vi "诊断标定3.vi"(8 "CAN端口":u16(ring), 9 "设备索引号":u16(ring), 10 "CAN卡类型":u32(ring)=21) -> ()   [LabVIEW 2013] (continued)
            n809 = property class="VI"(reference=w1301, error in=w1300, "Front Panel.Open"=FALSE ("前面板窗口:打开")) -> ()  [unwired: 2 out]
            n810 = call-poly <vilib>:"Write Key.vi"("section"="总信息", "error in (no error)"=w1293, "value"=w1288, "key"="诊断标定读取地址" ("section"), "refnum"=w1295) -> ("error out"=w1292:errorcluster, "refnum out"=w1291:T25)  [unwired: 4 in, 1 out]
            n811 = call <vilib>:"Close Config Data.vi"("error in (no error)"=w1292, "refnum"=w1291) -> ("error out"=w1290:errorcluster)  [unwired: 8 in, 1 out]
            n812 = call <vilib>:"Clear Errors.vi"("error in (no error)"=w1290) -> ()  [unwired: 6 in, 1 out]
            n813 = local write "强制终止读写标记"(TRUE ("强制终止读写标记")) -> ()
            n814 = local write "停止"(w1299) -> ()
          }
          frame #1 {
            w1307 = u8 0 items=["Normal", "Listen Only"] ("工作方式")
            w1308 = u8 1 items=["Dual Filter", "Single Filter"] ("滤波方式")
            n815 = local read "设备索引号"() -> (w1312:u16)
            n816 = local read "CAN卡类型"() -> (w1313:u32)
            n817 = local read "CAN端口"() -> (w1311:u16)
            n818 = call "CAN_Init-8.6.vi"("CAN卡类型"=w1313, "设备索引号"=w1312, "CAN端口"=w1311, "操作类型"=enum16{"初始化CAN", "关闭CAN"}."初始化CAN", "滤波方式"=w1308, "Accept Code"=u32 0, "簇"=T21 {"打开CAN"=FALSE, "初始化CAN"=TRUE, "开始CAN"=TRUE, "重启"=FALSE, "关闭CAN"=FALSE}, "Mask Code"=u32 4294967295 ("Accept Code"), "工作方式"=w1307, "是否滤波"=FALSE) -> ()  [unwired: 4 in, 6 out]
          }
        }
        n819 = event-data("Discard?"=w1286) -> ()  [unwired: 1 in, 1 out]
      }
      event "终止读写按钮": Value Change {
        n820 = event-data() -> ("NewVal"=w1314:bool)  [unwired: 6 out]
        n821 = case shown="真" w1314 {
          frame False {
          }
          frame True {
            n822 = local write "强制终止读写标记"(TRUE ("强制终止读写标记")) -> ()
          }
        }
      }
      event "1": Value Change {
        w1323 = FALSE ("1")
        n823 = event-data() -> ()  [unwired: 7 out]
        n824 = local write "主板2"(T8."项目信息" ("主从板")) -> ()
        n825 = Not(x=w1323) -> (.not. x?=w1322:bool)
        n826 = local write "1"(w1322) -> ()
        n827 = local write "1 2"(w1323) -> ()
        n828 = local write "1 3"(w1323) -> ()
        n829 = local write "1 4"(w1323) -> ()
        n830 = local write "1 5"(w1323) -> ()
        n831 = local write "1 11"(w1323) -> ()
        n832 = global read "功能码全局.vi" "主板监控2"() -> (w1321:bool[])
        n833 = Index Array(array=w1321, index=6 ("索引")) -> (element=w1316:bool)
        n834 = Select(t=0, s=w1316, f=1) -> (s? t:f=w1317:i32)
        n835 = property on="项目信息" class="Tbl (严格)"("Disabled"=w1317) -> ()  [unwired: 2 in, 2 out]
        n836 = property on="电池实际容量(A)" class="DigNum (严格)"("Disabled"=w1317) -> ()  [unwired: 2 in, 2 out]
        n837 = property on="使用者" class="DigNum (严格)"("Disabled"=w1317) -> ()  [unwired: 2 in, 2 out]
        n838 = property on="SOH(%)" class="DigNum (严格)"("Disabled"=w1317) -> ()  [unwired: 2 in, 2 out]
        n839 = property on="电池额定容量(A)" class="DigNum (严格)"("Disabled"=w1317) -> ()  [unwired: 2 in, 2 out]
        n840 = property on="SOC(%)" class="DigNum (严格)"("Disabled"=w1317) -> ()  [unwired: 2 in, 2 out]
        n841 = property on="项目信息2" class="Clust (严格)"("DisabledEnum"=w1317) -> ()  [unwired: 2 in, 2 out]
        n842 = property on="系统时钟" class="Str"("Disabled"=w1317) -> ()  [unwired: 2 in, 2 out]
        n843 = property on="配置文件版本" class="Str"("Disabled"=w1317) -> ()  [unwired: 2 in, 2 out]
        n844 = property on="车架(牌)号" class="Str"("Disabled"=w1317) -> ()  [unwired: 2 in, 2 out]
        n845 = property on="产品编号" class="Str"("Disabled"=w1317) -> ()  [unwired: 2 in, 2 out]
      }
      event "1 2": Value Change {
        w1334 = FALSE ("1")
        n846 = event-data() -> ()  [unwired: 7 out]
        n847 = local write "主板2"(T8."一级故障阀值" ("主从板")) -> ()
        n848 = Not(x=w1334) -> (.not. x?=w1333:bool)
        n849 = local write "1"(w1334) -> ()
        n850 = local write "1 2"(w1333) -> ()
        n851 = local write "1 3"(w1334) -> ()
        n852 = local write "1 4"(w1334) -> ()
        n853 = local write "1 5"(w1334) -> ()
        n854 = local write "1 11"(w1334) -> ()
        n855 = global read "功能码全局.vi" "主板监控2"() -> (w1332:bool[])
        n856 = Index Array(array=w1332, index=6 ("索引")) -> (element=w1327:bool)
        n857 = Select(t=0, s=w1327, f=1) -> (s? t:f=w1330:i32)
        n858 = property on="一级故障" class="Clust (严格)"("DisabledEnum"=w1330) -> ()  [unwired: 2 in, 2 out]
      }
      event "1 3": Value Change {
        w1345 = FALSE ("1")
        n859 = event-data() -> ()  [unwired: 7 out]
        n860 = local write "主板2"(T8."二级故障阀值" ("主从板")) -> ()
        n861 = Not(x=w1345) -> (.not. x?=w1344:bool)
        n862 = local write "1"(w1345) -> ()
        n863 = local write "1 2"(w1345) -> ()
        n864 = local write "1 3"(w1344) -> ()
        n865 = local write "1 4"(w1345) -> ()
        n866 = local write "1 5"(w1345) -> ()
        n867 = local write "1 11"(w1345) -> ()
        n868 = global read "功能码全局.vi" "主板监控2"() -> (w1343:bool[])
        n869 = Index Array(array=w1343, index=6 ("索引")) -> (element=w1339:bool)
        n870 = Select(t=0, s=w1339, f=1) -> (s? t:f=w1338:i32)
        n871 = property on="一级故障 2" class="Clust (严格)"("DisabledEnum"=w1338) -> ()  [unwired: 2 in, 2 out]
      }
      event "1 4": Value Change {
        w1356 = FALSE ("1")
        n872 = event-data() -> ()  [unwired: 7 out]
        n873 = local write "主板2"(T8."三级故障阀值" ("主从板")) -> ()
        n874 = Not(x=w1356) -> (.not. x?=w1355:bool)
        n875 = local write "1"(w1356) -> ()
        n876 = local write "1 2"(w1356) -> ()
        n877 = local write "1 3"(w1356) -> ()
        n878 = local write "1 4"(w1355) -> ()
        n879 = local write "1 5"(w1356) -> ()
        n880 = local write "1 11"(w1356) -> ()
        n881 = global read "功能码全局.vi" "主板监控2"() -> (w1354:bool[])
        n882 = Index Array(array=w1354, index=6 ("索引")) -> (element=w1349:bool)
        n883 = Select(t=0, s=w1349, f=1) -> (s? t:f=w1352:i32)
        n884 = property on="一级故障 3" class="Clust (严格)"("DisabledEnum"=w1352) -> ()  [unwired: 2 in, 2 out]
      }
      event "1 5": Value Change {
        w1367 = FALSE ("1")
        n885 = event-data() -> ()  [unwired: 7 out]
        n886 = local write "主板2"(T8."控制参数" ("主从板")) -> ()
        n887 = Not(x=w1367) -> (.not. x?=w1366:bool)
        n888 = local write "1"(w1367) -> ()
        n889 = local write "1 2"(w1367) -> ()
        n890 = local write "1 3"(w1367) -> ()
        n891 = local write "1 4"(w1367) -> ()
        n892 = local write "1 5"(w1366) -> ()
        n893 = local write "1 11"(w1367) -> ()
        n894 = global read "功能码全局.vi" "主板监控2"() -> (w1363:bool[])
        n895 = Index Array(array=w1363, index=6 ("索引")) -> (element=w1361:bool)
        n896 = Select(t=0, s=w1361, f=1) -> (s? t:f=w1360:i32)
        n897 = property on="风机开启温度" class="DigNum (严格)"("Disabled"=w1360) -> ()  [unwired: 2 in, 2 out]
        n898 = property on="风机关闭温度" class="DigNum (严格)"("Disabled"=w1360) -> ()  [unwired: 2 in, 2 out]
        n899 = property on="加热开启温度" class="DigNum (严格)"("Disabled"=w1360) -> ()  [unwired: 2 in, 2 out]
        n900 = property on="加热关闭温度" class="DigNum (严格)"("Disabled"=w1360) -> ()  [unwired: 2 in, 2 out]
        n901 = property on="风机开启温差" class="DigNum (严格)"("Disabled"=w1360) -> ()  [unwired: 2 in, 2 out]
        n902 = property on="风机关闭温差" class="DigNum (严格)"("Disabled"=w1360) -> ()  [unwired: 2 in, 2 out]
        n903 = property on="加热控制参数" class="Clust (严格)"("DisabledEnum"=w1360) -> ()  [unwired: 2 in, 2 out]
        n904 = property on="最大允许总电压" class="DigNum (严格)"("Disabled"=w1360) -> ()  [unwired: 2 in, 2 out]
        n905 = property on="最大允许充电温度" class="DigNum (严格)"("Disabled"=w1360) -> ()  [unwired: 2 in, 2 out]
        n906 = property on="最小允许充电温度" class="DigNum (严格)"("Disabled"=w1360) -> ()  [unwired: 2 in, 2 out]
        n907 = property on="电流步长" class="DigNum (严格)"("Disabled"=w1360) -> ()  [unwired: 2 in, 2 out]
        n908 = property on="最大允许单体电压" class="DigNum (严格)"("Disabled"=w1360) -> ()  [unwired: 2 in, 2 out]
        n909 = property on="最小允许单体电压" class="DigNum (严格)"("Disabled"=w1360) -> ()  [unwired: 2 in, 2 out]
        n910 = property on="最大允许充电电流" class="DigNum (严格)"("Disabled"=w1360) -> ()  [unwired: 2 in, 2 out]
        n911 = property on="最小允许充电电流" class="DigNum (严格)"("Disabled"=w1360) -> ()  [unwired: 2 in, 2 out]
      }
      event "1 11": Value Change {
        w1378 = FALSE ("1")
        n912 = event-data() -> ()  [unwired: 7 out]
        n913 = local write "主板2"(T8."电池信息" ("主从板")) -> ()
        n914 = Not(x=w1378) -> (.not. x?=w1377:bool)
        n915 = local write "1"(w1378) -> ()
        n916 = local write "1 2"(w1378) -> ()
        n917 = local write "1 3"(w1378) -> ()
        n918 = local write "1 4"(w1378) -> ()
        n919 = local write "1 5"(w1378) -> ()
        n920 = local write "1 11"(w1377) -> ()
        n921 = global read "功能码全局.vi" "主板监控2"() -> (w1373:bool[])
        n922 = Index Array(array=w1373, index=6 ("索引")) -> (element=w1371:bool)
        n923 = Select(t=0, s=w1371, f=1) -> (s? t:f=w1374:i32)
        n924 = property on="电池串联" class="DigNum (严格)"("Disabled"=w1374) -> ()  [unwired: 2 in, 2 out]
        n925 = property on="电池并联" class="DigNum (严格)"("Disabled"=w1374) -> ()  [unwired: 2 in, 2 out]
        n926 = property on="电池包额定容量" class="DigNum (严格)"("Disabled"=w1374) -> ()  [unwired: 2 in, 2 out]
        n927 = property on="电池包额定能量(kWh)" class="DigNum (严格)"("Disabled"=w1374) -> ()  [unwired: 2 in, 2 out]
        n928 = property on="电池包额定总电压" class="DigNum (严格)"("Disabled"=w1374) -> ()  [unwired: 2 in, 2 out]
        n929 = property on="实际容量" class="DigNum (严格)"("Disabled"=w1374) -> ()  [unwired: 2 in, 2 out]
        n930 = property on="电池包组号" class="Str"("Disabled"=w1374) -> ()  [unwired: 2 in, 2 out]
        n931 = property on="电池生产日期" class="Str"("Disabled"=w1374) -> ()  [unwired: 2 in, 2 out]
        n932 = property on="电池厂家" class="Str"("Disabled"=w1374) -> ()  [unwired: 2 in, 2 out]
        n933 = property on="电池类型" class="Str"("Disabled"=w1374) -> ()  [unwired: 2 in, 2 out]
        n934 = property on="累计充电总安时" class="DigNum (严格)"("Disabled"=w1374) -> ()  [unwired: 2 in, 2 out]
        n935 = property on="累计放电总安时" class="DigNum (严格)"("Disabled"=w1374) -> ()  [unwired: 2 in, 2 out]
        n936 = property on="电池放空次数" class="DigNum (严格)"("Disabled"=w1374) -> ()  [unwired: 2 in, 2 out]
        n937 = property on="电池充满次数" class="DigNum (严格)"("Disabled"=w1374) -> ()  [unwired: 2 in, 2 out]
        n938 = property on="电池充电次数" class="DigNum (严格)"("Disabled"=w1374) -> ()  [unwired: 2 in, 2 out]
        n939 = property on="电池信息" class="Clust (严格)"("DisabledEnum"=w1374) -> ()  [unwired: 2 in, 2 out]
      }
      event "1 6": Value Change {
        w1389 = FALSE ("1 6")
        n940 = event-data() -> ()  [unwired: 7 out]
        n941 = local write "等级 2"(T19."从板信息" ("等级 2")) -> ()
        n942 = global read "功能码全局.vi" "主板监控2"() -> (w1384:bool[])
        n943 = Not(x=w1389) -> (.not. x?=w1388:bool)
        n944 = local write "1 6"(w1388) -> ()
        n945 = local write "1 7"(w1389) -> ()
        n946 = local write "1 8"(w1389) -> ()
        n947 = local write "1 9"(w1389) -> ()
        n948 = local write "1 10"(w1389) -> ()
        n949 = Index Array(array=w1384, index=6 ("索引")) -> (element=w1382:bool)
        n950 = Select(t=0, s=w1382, f=1) -> (s? t:f=w1385:i32)
        n951 = property on="项目信息 2" class="Tbl (严格)"("Disabled"=w1385) -> ()  [unwired: 2 in, 2 out]
        n952 = property on="加热控制参数" class="Clust (严格)"("Disabled"=w1385) -> ()  [unwired: 2 in, 2 out]
      }
      event "1 7": Value Change {
        w1400 = FALSE ("1 6")
        n953 = event-data() -> ()  [unwired: 7 out]
        n954 = global read "功能码全局.vi" "主板监控2"() -> (w1398:bool[])
        n955 = Index Array(array=w1398, index=6 ("索引")) -> (element=w1393:bool)
        n956 = local write "等级 2"(T19."一级故障阀值" ("等级 2")) -> ()
        n957 = Select(t=0, s=w1393, f=1) -> (s? t:f=w1394:i32)
        n958 = property on="一级故障 6" class="Clust (严格)"("DisabledEnum"=w1394) -> ()  [unwired: 2 in, 2 out]
        n959 = Not(x=w1400) -> (.not. x?=w1399:bool)
        n960 = local write "1 6"(w1400) -> ()
        n961 = local write "1 7"(w1399) -> ()
        n962 = local write "1 8"(w1400) -> ()
        n963 = local write "1 9"(w1400) -> ()
        n964 = local write "1 10"(w1400) -> ()
      }
      event "1 8": Value Change {
        w1411 = FALSE ("1 6")
        n965 = event-data() -> ()  [unwired: 7 out]
        n966 = global read "功能码全局.vi" "主板监控2"() -> (w1409:bool[])
        n967 = Index Array(array=w1409, index=6 ("索引")) -> (element=w1404:bool)
        n968 = local write "等级 2"(T19."二级故障阀值" ("等级 2")) -> ()
        n969 = Select(t=0, s=w1404, f=1) -> (s? t:f=w1405:i32)
        n970 = Not(x=w1411) -> (.not. x?=w1410:bool)
        n971 = property on="一级故障 7" class="Clust (严格)"("DisabledEnum"=w1405) -> ()  [unwired: 2 in, 2 out]
        n972 = local write "1 6"(w1411) -> ()
        n973 = local write "1 7"(w1411) -> ()
        n974 = local write "1 8"(w1410) -> ()
        n975 = local write "1 9"(w1411) -> ()
        n976 = local write "1 10"(w1411) -> ()
      }
      event "1 9": Value Change {
        w1422 = FALSE ("1 6")
        n977 = event-data() -> ()  [unwired: 7 out]
        n978 = global read "功能码全局.vi" "主板监控2"() -> (w1420:bool[])
        n979 = Index Array(array=w1420, index=6 ("索引")) -> (element=w1415:bool)
        n980 = Select(t=0, s=w1415, f=1) -> (s? t:f=w1416:i32)
        n981 = local write "等级 2"(T19."三级故障阀值" ("等级 2")) -> ()
        n982 = property on="一级故障 8" class="Clust (严格)"("DisabledEnum"=w1416) -> ()  [unwired: 2 in, 2 out]
        n983 = Not(x=w1422) -> (.not. x?=w1421:bool)
        n984 = local write "1 6"(w1422) -> ()
        n985 = local write "1 7"(w1422) -> ()
        n986 = local write "1 8"(w1422) -> ()
        n987 = local write "1 9"(w1421) -> ()
        n988 = local write "1 10"(w1422) -> ()
      }
      event "1 10": Value Change {
        w1433 = FALSE ("1 6")
        n989 = event-data() -> ()  [unwired: 7 out]
        n990 = global read "功能码全局.vi" "主板监控2"() -> (w1431:bool[])
        n991 = Index Array(array=w1431, index=6 ("索引")) -> (element=w1426:bool)
        n992 = Select(t=0, s=w1426, f=1) -> (s? t:f=w1427:i32)
        n993 = local write "等级 2"(T19."快换参数" ("等级 2")) -> ()
        n994 = property on="电池组信息" class="Clust (严格)"("Disabled"=w1427) -> ()  [unwired: 2 in, 2 out]
        n995 = Not(x=w1433) -> (.not. x?=w1432:bool)
        n996 = local write "1 6"(w1433) -> ()
        n997 = local write "1 7"(w1433) -> ()
        n998 = local write "1 8"(w1433) -> ()
        n999 = local write "1 9"(w1433) -> ()
        n1000 = local write "1 10"(w1432) -> ()
      }
      event "1 12": Value Change {
        w1438 = FALSE ("1 6")
        n1001 = event-data() -> ()  [unwired: 7 out]
        n1002 = global read "功能码全局.vi" "主板监控2"() -> (w1445:bool[])
        n1003 = Index Array(array=w1445, index=6 ("索引")) -> (element=w1441:bool)
        n1004 = Select(t=0, s=w1441, f=1) -> (s? t:f=w1437:i32)
        n1005 = local write "等级 2"(T14."均衡参数" ("等级 2")) -> ()
        n1006 = property on="均衡参数" class="Clust (严格)"("DisabledEnum"=w1437) -> ()  [unwired: 2 in, 2 out]
        n1007 = Not(x=w1438) -> (.not. x?=w1439:bool)
        n1008 = local write "1 12"(w1439) -> ()
        n1009 = local write "1 6"(w1438) -> ()
        n1010 = local write "1 7"(w1438) -> ()
        n1011 = local write "1 8"(w1438) -> ()
        n1012 = local write "1 9"(w1438) -> ()
        n1013 = local write "1 10"(w1438) -> ()
      }
      event "主板选项": Mouse Down {
        n1014 = event-data() -> ("CtlRef"=w1461:refnum<vi>)  [unwired: 8 out]
        n1015 = global read "功能码全局.vi" "主板监控2"() -> (w1450:bool[])
        n1016 = property class="Tree (严格)"(reference=w1461) -> ("Value"=w1453:string)  [unwired: 1 in, 2 out]
        n1017 = Index Array(array=w1450, index=6 ("索引")) -> (element=w1448:bool)
        n1018 = case shown="\"二维码\"" w1453 {
          tunnel: [T8."项目信息" ("主从板") T8."项目信息" ("主从板") T8."项目信息" ("主从板") T8."项目信息" ("主从板") T8."项目信息" ("主从板") T8."项目信息" ("主从板") T8."项目信息" ("主从板") T8."项目信息" ("主从板") T8."项目信息" ("主从板") T8."项目信息" ("主从板") T8."项目信息" ("主从板") T8."项目信息" ("主从板") T8."项目信息" ("主从板") T8."项目信息" ("主从板") T8."项目信息" ("主从板") T8."项目信息" ("主从板") T8."二级故障阀值" ("主从板") T8."三级故障阀值" ("主从板") T8."一级故障阀值" ("主从板") T8."控制参数" ("主从板") T8."控制参数" ("主从板") T8."电池信息" ("主从板") T8."电池信息" ("主从板") T8."电池信息" ("主从板") T8."电池信息" ("主从板") T8."电池信息" ("主从板") T8."项目信息" ("主从板")] -> w1460
          tunnel: [w1471 w1478 w1493 w1508 w1525 w1565 w1599 w1646 w1684 w1734 w1769 w1783 w1798 w1813 w1828 w1842 w1855 w1869 w1882 w1896 w1910 w1923 w1937 w1951 w1965 w1979 w1983] -> w1459
          tunnel: [w1472 w1479 w1494 w1509 w1526 w1566 w1600 w1647 w1685 w1735 w1770 w1784 w1799 w1814 w1829 w1843 w1855 w1869 w1881 w1896 w1910 w1923 w1937 w1951 w1965 w1979 w1984] -> w1458
          tunnel: [w1472 w1479 w1494 w1509 w1526 w1566 w1600 w1647 w1685 w1735 w1770 w1784 w1799 w1814 w1829 w1843 w1856 w1869 w1882 w1896 w1910 w1923 w1937 w1951 w1965 w1979 w1984] -> w1457
          tunnel: [w1472 w1479 w1494 w1509 w1526 w1566 w1600 w1647 w1685 w1735 w1770 w1784 w1799 w1814 w1829 w1843 w1855 w1868 w1882 w1896 w1910 w1923 w1937 w1951 w1965 w1979 w1984] -> w1456
          tunnel: [w1472 w1479 w1494 w1509 w1526 w1566 w1600 w1647 w1685 w1735 w1770 w1784 w1799 w1814 w1829 w1843 w1855 w1869 w1882 w1895 w1909 w1923 w1937 w1951 w1965 w1979 w1984] -> w1455
          tunnel: [w1472 w1479 w1494 w1509 w1526 w1566 w1600 w1647 w1685 w1735 w1770 w1784 w1799 w1814 w1829 w1843 w1855 w1869 w1882 w1896 w1910 w1922 w1936 w1950 w1964 w1978 w1984] -> w1454
          tunnel: [w1464 FALSE w1489 w1504 w1517 w1557 w1590 w1637 w1676 w1727 w1764 w1778 w1792 w1806 w1821 w1837 w1851 w1864 w1877 w1891 w1904 w1918 w1931 w1945 w1959 w1973 FALSE] -> w1452
          tunnel: [w1464 TRUE w1486 w1501 w1516 w1556 w1591 w1638 w1675 w1726 w1763 w1777 w1791 w1807 w1822 w1836 w1850 w1863 w1876 w1890 w1903 w1917 w1930 w1944 w1958 w1972 FALSE] -> w1451
          tunnel: w1448 -> [w1469 _ w1483 w1498 w1513 w1552 w1587 w1634 w1672 w1724 w1760 w1774 w1788 w1803 w1818 w1833 w1847 w1860 w1873 w1887 w1900 w1914 w1927 w1941 w1955 w1969 _]
          frame "项目信息" {
            w1472 = FALSE
            n1019 = Select(t=0, s=w1469, f=1) -> (s? t:f=w1467:i32)
            n1020 = property on="项目信息" class="Tbl (严格)"("Disabled"=w1467) -> ()  [unwired: 2 in, 2 out]
            n1021 = property on="电池实际容量(A)" class="DigNum (严格)"("Disabled"=w1467) -> ()  [unwired: 2 in, 2 out]
            n1022 = property on="使用者" class="DigNum (严格)"("Disabled"=w1467) -> ()  [unwired: 2 in, 2 out]
            n1023 = property on="SOH(%)" class="DigNum (严格)"("Disabled"=w1467) -> ()  [unwired: 2 in, 2 out]
            n1024 = property on="从板个数" class="DigNum (严格)"("NumText.BGColor"=u32 6618880) -> ()  [unwired: 2 in, 2 out]
            n1025 = property on="电池额定容量(A)" class="DigNum (严格)"("Disabled"=w1467) -> ()  [unwired: 2 in, 2 out]
            n1026 = property on="SOC(%)" class="DigNum (严格)"("Disabled"=w1467) -> ()  [unwired: 2 in, 2 out]
            n1027 = property on="项目信息2" class="Clust (严格)"("DisabledEnum"=w1467) -> ()  [unwired: 2 in, 2 out]
            n1028 = property on="系统时钟" class="Str"("Disabled"=w1467) -> ()  [unwired: 2 in, 2 out]
            n1029 = property on="配置文件版本" class="Str"("Disabled"=w1467) -> ()  [unwired: 2 in, 2 out]
            n1030 = property on="车架(牌)号" class="Str"("Disabled"=w1467) -> ()  [unwired: 2 in, 2 out]
            n1031 = property on="产品编号" class="Str"("Disabled"=w1467) -> ()  [unwired: 2 in, 2 out]
            n1032 = local read "项目信息结果"() -> (w1465:bool)
            n1033 = Not(x=w1465) -> (.not. x?=w1464:bool)
            n1034 = Not(x=w1472) -> (.not. x?=w1471:bool)
          }
          frame "校正时钟" {
            w1475 = 2
            w1479 = FALSE
            n1035 = property on="从板个数" class="DigNum (严格)"("NumText.BGColor"=u32 13816530) -> ()  [unwired: 2 in, 2 out]
            n1036 = property on="项目信息" class="Tbl (严格)"("Disabled"=w1475) -> ()  [unwired: 2 in, 2 out]
            n1037 = property on="电池实际容量(A)" class="DigNum (严格)"("Disabled"=w1475) -> ()  [unwired: 2 in, 2 out]
            n1038 = property on="使用者" class="DigNum (严格)"("Disabled"=w1475) -> ()  [unwired: 2 in, 2 out]
            n1039 = property on="SOH(%)" class="DigNum (严格)"("Disabled"=w1475) -> ()  [unwired: 2 in, 2 out]
            n1040 = property on="电池额定容量(A)" class="DigNum (严格)"("Disabled"=w1475) -> ()  [unwired: 2 in, 2 out]
            n1041 = property on="SOC(%)" class="DigNum (严格)"("Disabled"=w1475) -> ()  [unwired: 2 in, 2 out]
            n1042 = property on="系统时钟" class="Str"("Disabled"=w1475) -> ()  [unwired: 2 in, 2 out]
            n1043 = property on="配置文件版本" class="Str"("Disabled"=w1475) -> ()  [unwired: 2 in, 2 out]
            n1044 = property on="车架(牌)号" class="Str"("Disabled"=w1475) -> ()  [unwired: 2 in, 2 out]
            n1045 = property on="项目信息2" class="Clust (严格)"("DisabledEnum"=w1475) -> ()  [unwired: 2 in, 2 out]
            n1046 = property on="产品编号" class="Str"("Disabled"=w1475) -> ()  [unwired: 2 in, 2 out]
            n1047 = Not(x=w1479) -> (.not. x?=w1478:bool)
          }
          frame "产品编号" {
            w1492 = 2
            w1494 = FALSE
            n1048 = property on="项目信息" class="Tbl (严格)"("Disabled"=w1492) -> ()  [unwired: 2 in, 2 out]
            n1049 = property on="电池实际容量(A)" class="DigNum (严格)"("Disabled"=w1492) -> ()  [unwired: 2 in, 2 out]
            n1050 = property on="使用者" class="DigNum (严格)"("Disabled"=w1492) -> ()  [unwired: 2 in, 2 out]
            n1051 = Select(t=0, s=w1483, f=1) -> (s? t:f=w1482:i32)
            n1052 = property on="SOH(%)" class="DigNum (严格)"("Disabled"=w1492) -> ()  [unwired: 2 in, 2 out]
            n1053 = property on="电池额定容量(A)" class="DigNum (严格)"("Disabled"=w1492) -> ()  [unwired: 2 in, 2 out]
            n1054 = property on="SOC(%)" class="DigNum (严格)"("Disabled"=w1492) -> ()  [unwired: 2 in, 2 out]
            n1055 = property on="产品编号" class="Str"("Disabled"=w1482) -> ()  [unwired: 2 in, 2 out]
            n1056 = property on="项目信息2" class="Clust (严格)"("DisabledEnum"=w1482) -> ()  [unwired: 2 in, 2 out]
            n1057 = property on="系统时钟" class="Str"("Disabled"=w1492) -> ()  [unwired: 2 in, 2 out]
            n1058 = property on="配置文件版本" class="Str"("Disabled"=w1492) -> ()  [unwired: 2 in, 2 out]
            n1059 = property on="车架(牌)号" class="Str"("Disabled"=w1492) -> ()  [unwired: 2 in, 2 out]
            n1060 = property on="从板个数" class="DigNum (严格)"("NumText.BGColor"=u32 13816530) -> ()  [unwired: 2 in, 2 out]
            n1061 = global read "功能码全局.vi" "主板项目信息5"() -> (w1490:bool[])
            n1062 = global read "功能码全局.vi" "主板项目信息6"() -> (w1487:bool[])
            n1063 = Index Array(array=w1490, index=0 ("索引")) -> (element=w1489:bool)
            n1064 = Index Array(array=w1487, index=1 ("索引")) -> (element=w1486:bool)
            n1065 = Not(x=w1494) -> (.not. x?=w1493:bool)
          }
          frame "二维码" {
            w1507 = 2
            w1509 = FALSE
            n1066 = property on="项目信息" class="Tbl (严格)"("Disabled"=w1507) -> ()  [unwired: 2 in, 2 out]
            n1067 = property on="电池实际容量(A)" class="DigNum (严格)"("Disabled"=w1507) -> ()  [unwired: 2 in, 2 out]
            n1068 = property on="使用者" class="DigNum (严格)"("Disabled"=w1507) -> ()  [unwired: 2 in, 2 out]
            n1069 = Select(t=0, s=w1498, f=1) -> (s? t:f=w1497:i32)
            n1070 = property on="SOH(%)" class="DigNum (严格)"("Disabled"=w1507) -> ()  [unwired: 2 in, 2 out]
            n1071 = property on="电池额定容量(A)" class="DigNum (严格)"("Disabled"=w1507) -> ()  [unwired: 2 in, 2 out]
            n1072 = property on="SOC(%)" class="DigNum (严格)"("Disabled"=w1507) -> ()  [unwired: 2 in, 2 out]
            n1073 = property on="产品编号" class="Str"("Disabled"=w1497) -> ()  [unwired: 2 in, 2 out]
            n1074 = property on="项目信息2" class="Clust (严格)"("DisabledEnum"=w1497) -> ()  [unwired: 2 in, 2 out]
            n1075 = property on="系统时钟" class="Str"("Disabled"=w1507) -> ()  [unwired: 2 in, 2 out]
            n1076 = property on="配置文件版本" class="Str"("Disabled"=w1507) -> ()  [unwired: 2 in, 2 out]
            n1077 = property on="车架(牌)号" class="Str"("Disabled"=w1507) -> ()  [unwired: 2 in, 2 out]
            n1078 = property on="从板个数" class="DigNum (严格)"("NumText.BGColor"=u32 13816530) -> ()  [unwired: 2 in, 2 out]
            n1079 = global read "功能码全局.vi" "主板项目信息5"() -> (w1505:bool[])
            n1080 = global read "功能码全局.vi" "主板项目信息6"() -> (w1502:bool[])
            n1081 = Index Array(array=w1505, index=0 ("索引")) -> (element=w1504:bool)
            n1082 = Index Array(array=w1502, index=1 ("索引")) -> (element=w1501:bool)
            n1083 = Not(x=w1509) -> (.not. x?=w1508:bool)
          }
          frame "电压个数" {
            w1524 = 2
            w1526 = FALSE
            n1084 = local read "从板个数"() -> (w1523:dbl)
            n1085 = property on="从板个数" class="DigNum (严格)"("NumText.BGColor"=u32 6618880) -> ()  [unwired: 2 in, 2 out]
            n1086 = property on="电池实际容量(A)" class="DigNum (严格)"("Disabled"=w1524) -> ()  [unwired: 2 in, 2 out]
            n1087 = property on="使用者" class="DigNum (严格)"("Disabled"=w1524) -> ()  [unwired: 2 in, 2 out]
            n1088 = property on="SOH(%)" class="DigNum (严格)"("Disabled"=w1524) -> ()  [unwired: 2 in, 2 out]
            n1089 = property on="电池额定容量(A)" class="DigNum (严格)"("Disabled"=w1524) -> ()  [unwired: 2 in, 2 out]
            n1090 = property on="SOC(%)" class="DigNum (严格)"("Disabled"=w1524) -> ()  [unwired: 2 in, 2 out]
            n1091 = property on="系统时钟" class="Str"("Disabled"=w1524) -> ()  [unwired: 2 in, 2 out]
            n1092 = property on="配置文件版本" class="Str"("Disabled"=w1524) -> ()  [unwired: 2 in, 2 out]
            n1093 = property on="车架(牌)号" class="Str"("Disabled"=w1524) -> ()  [unwired: 2 in, 2 out]
            n1094 = property on="产品编号" class="Str"("Disabled"=w1524) -> ()  [unwired: 2 in, 2 out]
            n1095 = Select(t=0, s=w1513, f=1) -> (s? t:f=w1512:i32)
            n1096 = control-ref of="项目信息"() -> (w1522:refnum<vi>)
            n1097 = stacked-sequence {
              tunnel: w1523 -> [_ w1533 w1543]
              tunnel: w1522 -> [w1528 w1532 w1544]
              frame #0 {
                w1529 = 0
                n1098 = Bundle(w1529, w1529) -> (w1531:cluster{i32, i32})  [unwired: 1 out]
                n1099 = property class="Tbl (严格)"(reference=w1528, "Index Values"=w1531) -> (error out=w1530:errorcluster)  [unwired: 1 in, 1 out]
                n1100 = call <vilib>:"Clear Errors.vi"("error in (no error)"=w1530) -> ()  [unwired: 7 out]
              }
              frame #1 {
                n1101 = for {
                  N: 10 -> [_]
                  tunnel: w1532 -> [w1542]
                  tunnel: w1533 -> [w1537]
                  i -> [w1536]
                  n1102 = Compound Arithmetic op=ADD(0.0 ("值"), w1537, w1536) -> (w1539:dbl)
                  n1103 = Bundle(w1539, 0) -> (w1541:cluster{dbl, i32})  [unwired: 1 out]
                  n1104 = property class="Tbl (严格)"(reference=w1542, "Active Cell"=w1541, "Cell BG Color"=u32 16448250) -> ()  [unwired: 1 in, 2 out]
                }
              }
              frame #2 {
                n1105 = for {
                  N: w1543 -> [_]
                  tunnel: w1544 -> [w1545]
                  i -> [w1546]
                  n1106 = Bundle(w1546, 0) -> (w1550:cluster{i32, i32})  [unwired: 1 out]
                  n1107 = property class="Tbl (严格)"(reference=w1545, "Active Cell"=w1550, "Cell BG Color"=u32 6618880) -> (error out=w1547:errorcluster)  [unwired: 1 in, 1 out]
                  n1108 = call <vilib>:"Clear Errors.vi"("error in (no error)"=w1547) -> ()  [unwired: 7 out]
                }
              }
            }
            n1109 = property on="项目信息" class="Tbl (严格)"("Disabled"=w1512) -> ()  [unwired: 2 in, 2 out]
            n1110 = global read "功能码全局.vi" "主板项目信息5"() -> (w1520:bool[])
            n1111 = global read "功能码全局.vi" "主板项目信息6"() -> (w1518:bool[])
            n1112 = Index Array(array=w1520, index=1 ("索引")) -> (element=w1517:bool)
            n1113 = Index Array(array=w1518, index=2 ("索引")) -> (element=w1516:bool)
            n1114 = Not(x=w1526) -> (.not. x?=w1525:bool)
          }
          frame "通道电压数" {
            w1564 = 2
            w1566 = FALSE
            n1115 = property on="从板个数" class="DigNum (严格)"("NumText.BGColor"=u32 13816530) -> ()  [unwired: 2 in, 2 out]
            n1116 = property on="电池实际容量(A)" class="DigNum (严格)"("Disabled"=w1564) -> ()  [unwired: 2 in, 2 out]
            n1117 = property on="使用者" class="DigNum (严格)"("Disabled"=w1564) -> ()  [unwired: 2 in, 2 out]
            n1118 = property on="SOH(%)" class="DigNum (严格)"("Disabled"=w1564) -> ()  [unwired: 2 in, 2 out]
            n1119 = property on="电池额定容量(A)" class="DigNum (严格)"("Disabled"=w1564) -> ()  [unwired: 2 in, 2 out]
            n1120 = property on="SOC(%)" class="DigNum (严格)"("Disabled"=w1564) -> ()  [unwired: 2 in, 2 out]
            n1121 = local read "从板个数"() -> (w1562:dbl)
            n1122 = property on="系统时钟" class="Str"("Disabled"=w1564) -> ()  [unwired: 2 in, 2 out]
            n1123 = property on="配置文件版本" class="Str"("Disabled"=w1564) -> ()  [unwired: 2 in, 2 out]
            n1124 = property on="车架(牌)号" class="Str"("Disabled"=w1564) -> ()  [unwired: 2 in, 2 out]
            n1125 = property on="产品编号" class="Str"("Disabled"=w1564) -> ()  [unwired: 2 in, 2 out]
            n1126 = control-ref of="项目信息"() -> (w1563:refnum<vi>)
            n1127 = stacked-sequence {
              tunnel: w1563 -> [w1573 w1576]
              tunnel: w1562 -> [w1572 w1575]
              frame #0 {
                n1128 = Compound Arithmetic op=ADD(1.0 ("值"), w1572) -> (w1569:dbl)
                n1129 = Bundle(w1569, 0) -> (w1571:cluster{dbl, i32})  [unwired: 1 out]
                n1130 = property class="Tbl (严格)"(reference=w1573, "Index Values"=w1571) -> ()  [unwired: 1 in, 2 out]
              }
              frame #1 {
                n1131 = for {
                  N: 20 -> [_]
                  tunnel: w1576 -> [w1584]
                  tunnel: w1575 -> [w1579]
                  i -> [w1578]
                  n1132 = Compound Arithmetic op=ADD(1.0 ("值"), w1579, w1578) -> (w1581:dbl)
                  n1133 = Bundle(w1581, 0) -> (w1583:cluster{dbl, i32})  [unwired: 1 out]
                  n1134 = property class="Tbl (严格)"(reference=w1584, "Active Cell"=w1583, "Cell BG Color"=u32 6618880) -> ()  [unwired: 1 in, 2 out]
                }
              }
            }
            n1135 = Select(t=0, s=w1552, f=1) -> (s? t:f=w1553:i32)
            n1136 = property on="项目信息" class="Tbl (严格)"("Disabled"=w1553) -> ()  [unwired: 2 in, 2 out]
            n1137 = global read "功能码全局.vi" "主板项目信息5"() -> (w1560:bool[])
            n1138 = global read "功能码全局.vi" "主板项目信息6"() -> (w1558:bool[])
            n1139 = Index Array(array=w1560, index=2 ("索引")) -> (element=w1557:bool)
            n1140 = Index Array(array=w1558, index=3 ("索引")) -> (element=w1556:bool)
            n1141 = Not(x=w1566) -> (.not. x?=w1565:bool)
          }
          frame "电压起始值" {
            w1598 = 2
            w1600 = FALSE
            n1142 = property on="从板个数" class="DigNum (严格)"("NumText.BGColor"=u32 13816530) -> ()  [unwired: 2 in, 2 out]
            n1143 = property on="电池实际容量(A)" class="DigNum (严格)"("Disabled"=w1598) -> ()  [unwired: 2 in, 2 out]
            n1144 = property on="使用者" class="DigNum (严格)"("Disabled"=w1598) -> ()  [unwired: 2 in, 2 out]
            n1145 = property on="SOH(%)" class="DigNum (严格)"("Disabled"=w1598) -> ()  [unwired: 2 in, 2 out]
            n1146 = property on="电池额定容量(A)" class="DigNum (严格)"("Disabled"=w1598) -> ()  [unwired: 2 in, 2 out]
            n1147 = property on="SOC(%)" class="DigNum (严格)"("Disabled"=w1598) -> ()  [unwired: 2 in, 2 out]
            n1148 = local read "从板个数"() -> (w1596:dbl)
            n1149 = property on="系统时钟" class="Str"("Disabled"=w1598) -> ()  [unwired: 2 in, 2 out]
            n1150 = property on="配置文件版本" class="Str"("Disabled"=w1598) -> ()  [unwired: 2 in, 2 out]
            n1151 = property on="车架(牌)号" class="Str"("Disabled"=w1598) -> ()  [unwired: 2 in, 2 out]
            n1152 = property on="产品编号" class="Str"("Disabled"=w1598) -> ()  [unwired: 2 in, 2 out]
            n1153 = control-ref of="项目信息"() -> (w1597:refnum<vi>)
            n1154 = stacked-sequence {
              tunnel: w1597 -> [w1607 w1610 w1623]
              tunnel: w1596 -> [w1606 w1609 w1622]
              frame #0 {
                n1155 = Compound Arithmetic op=ADD(21.0 ("值"), w1606) -> (w1603:dbl)
                n1156 = Bundle(w1603, 0) -> (w1605:cluster{dbl, i32})  [unwired: 1 out]
                n1157 = property class="Tbl (严格)"(reference=w1607, "Index Values"=w1605) -> ()  [unwired: 1 in, 2 out]
              }
              frame #1 {
                n1158 = for {
                  N: 10 -> [_]
                  tunnel: w1610 -> [w1620]
                  tunnel: w1609 -> [w1615]
                  i -> [w1614]
                  n1159 = Multiply(x=w1615, y=2.0) -> (x*y=w1612:dbl)
                  n1160 = Compound Arithmetic op=ADD(21.0 ("值"), w1612, w1614) -> (w1617:dbl)
                  n1161 = Bundle(w1617, 0) -> (w1619:cluster{dbl, i32})  [unwired: 1 out]
                  n1162 = property class="Tbl (严格)"(reference=w1620, "Active Cell"=w1619, "Cell BG Color"=u32 16448250) -> ()  [unwired: 1 in, 2 out]
                }
              }
              frame #2 {
                n1163 = Increment(x=w1622) -> (x+1=w1621:dbl)
                n1164 = for {
                  N: w1621 -> [_]
                  tunnel: w1623 -> [w1631]
                  tunnel: w1622 -> [w1626]
                  i -> [w1625]
                  n1165 = Compound Arithmetic op=ADD(21.0 ("值"), w1626, w1625) -> (w1628:dbl)
                  n1166 = Bundle(w1628, 0) -> (w1630:cluster{dbl, i32})  [unwired: 1 out]
                  n1167 = property class="Tbl (严格)"(reference=w1631, "Active Cell"=w1630, "Cell BG Color"=u32 6618880) -> ()  [unwired: 1 in, 2 out]
                }
              }
            }
            n1168 = Select(t=0, s=w1587, f=1) -> (s? t:f=w1586:i32)
            n1169 = property on="项目信息" class="Tbl (严格)"("Disabled"=w1586) -> ()  [unwired: 2 in, 2 out]
            n1170 = global read "功能码全局.vi" "主板项目信息5"() -> (w1594:bool[])
            n1171 = global read "功能码全局.vi" "主板项目信息6"() -> (w1592:bool[])
            n1172 = Index Array(array=w1594, index=3 ("索引")) -> (element=w1590:bool)
            n1173 = Index Array(array=w1592, index=4 ("索引")) -> (element=w1591:bool)
            n1174 = Not(x=w1600) -> (.not. x?=w1599:bool)
          }
          frame "温度个数" {
            w1645 = 2
            w1647 = FALSE
            n1175 = property on="电池实际容量(A)" class="DigNum (严格)"("Disabled"=w1645) -> ()  [unwired: 2 in, 2 out]
            n1176 = property on="使用者" class="DigNum (严格)"("Disabled"=w1645) -> ()  [unwired: 2 in, 2 out]
            n1177 = property on="SOH(%)" class="DigNum (严格)"("Disabled"=w1645) -> ()  [unwired: 2 in, 2 out]
            n1178 = property on="电池额定容量(A)" class="DigNum (严格)"("Disabled"=w1645) -> ()  [unwired: 2 in, 2 out]
            n1179 = property on="SOC(%)" class="DigNum (严格)"("Disabled"=w1645) -> ()  [unwired: 2 in, 2 out]
            n1180 = local read "从板个数"() -> (w1643:dbl)
            n1181 = control-ref of="项目信息"() -> (w1644:refnum<vi>)
            n1182 = stacked-sequence {
              tunnel: w1644 -> [w1652 w1655 w1662]
              tunnel: w1643 -> [w1649 w1654 w1661]
              frame #0 {
                n1183 = Bundle("从板个数"=w1649, 0) -> (w1651:cluster{"从板个数":dbl, i32})  [unwired: 1 out]
                n1184 = property class="Tbl (严格)"(reference=w1652, "Index Values"=w1651) -> ()  [unwired: 1 in, 2 out]
              }
              frame #1 {
                n1185 = for {
                  N: 20 -> [_]
                  tunnel: w1655 -> [w1660]
                  tunnel: w1654 -> [_]
                  i -> [w1656]
                  n1186 = Bundle(w1656, 0) -> (w1659:cluster{i32, i32})  [unwired: 1 out]
                  n1187 = property class="Tbl (严格)"(reference=w1660, "Active Cell"=w1659, "Cell BG Color"=u32 16448250) -> ()  [unwired: 1 in, 2 out]
                }
              }
              frame #2 {
                n1188 = for {
                  N: w1661 -> [_]
                  tunnel: w1662 -> [w1669]
                  tunnel: w1661 -> [w1663]
                  i -> [w1664]
                  n1189 = Compound Arithmetic op=ADD(w1663, w1664) -> (w1666:dbl)
                  n1190 = Bundle(w1666, 0) -> (w1668:cluster{dbl, i32})  [unwired: 1 out]
                  n1191 = property class="Tbl (严格)"(reference=w1669, "Active Cell"=w1668, "Cell BG Color"=u32 6618880) -> ()  [unwired: 1 in, 2 out]
                }
              }
            }
            n1192 = property on="系统时钟" class="Str"("Disabled"=w1645) -> ()  [unwired: 2 in, 2 out]
            n1193 = property on="配置文件版本" class="Str"("Disabled"=w1645) -> ()  [unwired: 2 in, 2 out]
            n1194 = property on="车架(牌)号" class="Str"("Disabled"=w1645) -> ()  [unwired: 2 in, 2 out]
            n1195 = property on="产品编号" class="Str"("Disabled"=w1645) -> ()  [unwired: 2 in, 2 out]
            n1196 = property on="从板个数" class="DigNum (严格)"("NumText.BGColor"=u32 13816530) -> ()  [unwired: 2 in, 2 out]
            n1197 = Select(t=0, s=w1634, f=1) -> (s? t:f=w1633:i32)
            n1198 = property on="项目信息" class="Tbl (严格)"("Disabled"=w1633) -> ()  [unwired: 2 in, 2 out]
            n1199 = global read "功能码全局.vi" "主板项目信息5"() -> (w1641:bool[])
            n1200 = global read "功能码全局.vi" "主板项目信息6"() -> (w1639:bool[])
            n1201 = Index Array(array=w1641, index=4 ("索引")) -> (element=w1637:bool)
            n1202 = Index Array(array=w1639, index=5 ("索引")) -> (element=w1638:bool)
            n1203 = Not(x=w1647) -> (.not. x?=w1646:bool)
          }
          frame "温度起始值" {
            w1683 = 2
            w1685 = FALSE
            n1204 = property on="电池实际容量(A)" class="DigNum (严格)"("Disabled"=w1683) -> ()  [unwired: 2 in, 2 out]
            n1205 = property on="使用者" class="DigNum (严格)"("Disabled"=w1683) -> ()  [unwired: 2 in, 2 out]
            n1206 = property on="SOH(%)" class="DigNum (严格)"("Disabled"=w1683) -> ()  [unwired: 2 in, 2 out]
            n1207 = property on="电池额定容量(A)" class="DigNum (严格)"("Disabled"=w1683) -> ()  [unwired: 2 in, 2 out]
            n1208 = property on="SOC(%)" class="DigNum (严格)"("Disabled"=w1683) -> ()  [unwired: 2 in, 2 out]
            n1209 = local read "从板个数"() -> (w1681:dbl)
            n1210 = property on="系统时钟" class="Str"("Disabled"=w1683) -> ()  [unwired: 2 in, 2 out]
            n1211 = property on="配置文件版本" class="Str"("Disabled"=w1683) -> ()  [unwired: 2 in, 2 out]
            n1212 = property on="车架(牌)号" class="Str"("Disabled"=w1683) -> ()  [unwired: 2 in, 2 out]
            n1213 = property on="产品编号" class="Str"("Disabled"=w1683) -> ()  [unwired: 2 in, 2 out]
            n1214 = control-ref of="项目信息"() -> (w1682:refnum<vi>)
            n1215 = stacked-sequence {
              tunnel: w1682 -> [w1694 w1697 w1710]
              tunnel: w1681 -> [w1687 w1696 w1709]
              frame #0 {
                n1216 = Multiply(x=w1687, y=3.0) -> (x*y=w1689:dbl)
                n1217 = Compound Arithmetic op=ADD(23.0 ("值"), w1689) -> (w1691:dbl)
                n1218 = Bundle(w1691, 0) -> (w1693:cluster{dbl, i32})  [unwired: 1 out]
                n1219 = property class="Tbl (严格)"(reference=w1694, "Index Values"=w1693) -> ()  [unwired: 1 in, 2 out]
              }
              frame #1 {
                n1220 = for {
                  N: 10 -> [_]
                  tunnel: w1697 -> [w1707]
                  tunnel: w1696 -> [w1702]
                  i -> [w1701]
                  n1221 = Multiply(x=4.0, y=w1702) -> (x*y=w1699:dbl)
                  n1222 = Compound Arithmetic op=ADD(24.0 ("值"), w1699, w1701) -> (w1704:dbl)
                  n1223 = Bundle(w1704, 0) -> (w1706:cluster{dbl, i32})  [unwired: 1 out]
                  n1224 = property class="Tbl (严格)"(reference=w1707, "Active Cell"=w1706, "Cell BG Color"=u32 16448250) -> ()  [unwired: 1 in, 2 out]
                }
              }
              frame #2 {
                n1225 = Increment(x=w1709) -> (x+1=w1708:dbl)
                n1226 = for {
                  N: w1708 -> [_]
                  tunnel: w1710 -> [w1720]
                  tunnel: w1709 -> [w1715]
                  i -> [w1714]
                  n1227 = Multiply(x=3.0, y=w1715) -> (x*y=w1712:dbl)
                  n1228 = Compound Arithmetic op=ADD(23.0 ("值"), w1712, w1714) -> (w1717:dbl)
                  n1229 = Bundle(w1717, 0) -> (w1719:cluster{dbl, i32})  [unwired: 1 out]
                  n1230 = property class="Tbl (严格)"(reference=w1720, "Active Cell"=w1719, "Cell BG Color"=u32 6618880) -> ()  [unwired: 1 in, 2 out]
                }
              }
            }
            n1231 = Select(t=0, s=w1672, f=1) -> (s? t:f=w1671:i32)
            n1232 = property on="从板个数" class="DigNum (严格)"("NumText.BGColor"=u32 13816530) -> ()  [unwired: 2 in, 2 out]
            n1233 = property on="项目信息" class="Tbl (严格)"("Disabled"=w1671) -> ()  [unwired: 2 in, 2 out]
            n1234 = global read "功能码全局.vi" "主板项目信息5"() -> (w1679:bool[])
            n1235 = global read "功能码全局.vi" "主板项目信息6"() -> (w1677:bool[])
            n1236 = Index Array(array=w1679, index=5 ("索引")) -> (element=w1676:bool)
            n1237 = Index Array(array=w1677, index=6 ("索引")) -> (element=w1675:bool)
            n1238 = Not(x=w1685) -> (.not. x?=w1684:bool)
          }
          frame "保险位置" {
            w1733 = 2
            w1735 = FALSE
            n1239 = property on="电池实际容量(A)" class="DigNum (严格)"("Disabled"=w1733) -> ()  [unwired: 2 in, 2 out]
            n1240 = property on="使用者" class="DigNum (严格)"("Disabled"=w1733) -> ()  [unwired: 2 in, 2 out]
            n1241 = property on="SOH(%)" class="DigNum (严格)"("Disabled"=w1733) -> ()  [unwired: 2 in, 2 out]
            n1242 = property on="电池额定容量(A)" class="DigNum (严格)"("Disabled"=w1733) -> ()  [unwired: 2 in, 2 out]
            n1243 = property on="SOC(%)" class="DigNum (严格)"("Disabled"=w1733) -> ()  [unwired: 2 in, 2 out]
            n1244 = local read "从板个数"() -> (w1731:dbl)
            n1245 = property on="系统时钟" class="Str"("Disabled"=w1733) -> ()  [unwired: 2 in, 2 out]
            n1246 = property on="配置文件版本" class="Str"("Disabled"=w1733) -> ()  [unwired: 2 in, 2 out]
            n1247 = property on="车架(牌)号" class="Str"("Disabled"=w1733) -> ()  [unwired: 2 in, 2 out]
            n1248 = property on="产品编号" class="Str"("Disabled"=w1733) -> ()  [unwired: 2 in, 2 out]
            n1249 = control-ref of="项目信息"() -> (w1732:refnum<vi>)
            n1250 = stacked-sequence {
              tunnel: w1732 -> [w1744 w1747]
              tunnel: w1731 -> [w1737 w1746]
              frame #0 {
                n1251 = Multiply(x=w1737, y=4.0) -> (x*y=w1739:dbl)
                n1252 = Compound Arithmetic op=ADD(24.0 ("值"), w1739) -> (w1741:dbl)
                n1253 = Bundle(w1741, 0) -> (w1743:cluster{dbl, i32})  [unwired: 1 out]
                n1254 = property class="Tbl (严格)"(reference=w1744, "Index Values"=w1743) -> ()  [unwired: 1 in, 2 out]
              }
              frame #1 {
                n1255 = for {
                  N: 20 -> [_]
                  tunnel: w1747 -> [w1757]
                  tunnel: w1746 -> [w1752]
                  i -> [w1751]
                  n1256 = Multiply(x=4.0, y=w1752) -> (x*y=w1749:dbl)
                  n1257 = Compound Arithmetic op=ADD(24.0 ("值"), w1749, w1751) -> (w1754:dbl)
                  n1258 = Bundle(w1754, 0) -> (w1756:cluster{dbl, i32})  [unwired: 1 out]
                  n1259 = property class="Tbl (严格)"(reference=w1757, "Active Cell"=w1756, "Cell BG Color"=u32 6618880) -> ()  [unwired: 1 in, 2 out]
                }
              }
            }
            n1260 = property on="从板个数" class="DigNum (严格)"("NumText.BGColor"=u32 13816530) -> ()  [unwired: 2 in, 2 out]
            n1261 = Select(t=0, s=w1724, f=1) -> (s? t:f=w1722:i32)
            n1262 = global read "功能码全局.vi" "主板项目信息4"() -> (w1729:bool[])
            n1263 = property on="项目信息" class="Tbl (严格)"("Disabled"=w1722) -> ()  [unwired: 2 in, 2 out]
            n1264 = Index Array(array=w1729, index #1=5 ("索引"), index #2=6 ("索引")) -> (element #1=w1727:bool, element #2=w1726:bool)
            n1265 = Not(x=w1735) -> (.not. x?=w1734:bool)
          }
          frame "SOC" {
            w1768 = 2
            w1770 = FALSE
            n1266 = property on="电池实际容量(A)" class="DigNum (严格)"("Disabled"=w1768) -> ()  [unwired: 2 in, 2 out]
            n1267 = property on="使用者" class="DigNum (严格)"("Disabled"=w1768) -> ()  [unwired: 2 in, 2 out]
            n1268 = property on="SOH(%)" class="DigNum (严格)"("Disabled"=w1768) -> ()  [unwired: 2 in, 2 out]
            n1269 = property on="电池额定容量(A)" class="DigNum (严格)"("Disabled"=w1768) -> ()  [unwired: 2 in, 2 out]
            n1270 = property on="从板个数" class="DigNum (严格)"("NumText.BGColor"=u32 13816530) -> ()  [unwired: 2 in, 2 out]
            n1271 = property on="系统时钟" class="Str"("Disabled"=w1768) -> ()  [unwired: 2 in, 2 out]
            n1272 = property on="配置文件版本" class="Str"("Disabled"=w1768) -> ()  [unwired: 2 in, 2 out]
            n1273 = property on="车架(牌)号" class="Str"("Disabled"=w1768) -> ()  [unwired: 2 in, 2 out]
            n1274 = property on="项目信息" class="Tbl (严格)"("Disabled"=w1768) -> ()  [unwired: 2 in, 2 out]
            n1275 = property on="产品编号" class="Str"("Disabled"=w1768) -> ()  [unwired: 2 in, 2 out]
            n1276 = Select(t=0, s=w1760, f=0) -> (s? t:f=w1759:i32)
            n1277 = property on="SOC(%)" class="DigNum (严格)"("Disabled"=w1759) -> ()  [unwired: 2 in, 2 out]
            n1278 = property on="项目信息2" class="Clust (严格)"("DisabledEnum"=w1759) -> ()  [unwired: 2 in, 2 out]
            n1279 = global read "功能码全局.vi" "主板项目信息7"() -> (w1766:bool[])
            n1280 = Index Array(array=w1766, index #1=2 ("索引"), index #2=5 ("索引")) -> (element #1=w1764:bool, element #2=w1763:bool)
            n1281 = Not(x=w1770) -> (.not. x?=w1769:bool)
          }
          frame "电池额定实际容量" {
            w1782 = 2
            w1784 = FALSE
            n1282 = property on="使用者" class="DigNum (严格)"("Disabled"=w1782) -> ()  [unwired: 2 in, 2 out]
            n1283 = property on="SOH(%)" class="DigNum (严格)"("Disabled"=w1782) -> ()  [unwired: 2 in, 2 out]
            n1284 = property on="SOC(%)" class="DigNum (严格)"("Disabled"=w1782) -> ()  [unwired: 2 in, 2 out]
            n1285 = property on="从板个数" class="DigNum (严格)"("NumText.BGColor"=u32 13816530) -> ()  [unwired: 2 in, 2 out]
            n1286 = property on="系统时钟" class="Str"("Disabled"=w1782) -> ()  [unwired: 2 in, 2 out]
            n1287 = property on="配置文件版本" class="Str"("Disabled"=w1782) -> ()  [unwired: 2 in, 2 out]
            n1288 = property on="车架(牌)号" class="Str"("Disabled"=w1782) -> ()  [unwired: 2 in, 2 out]
            n1289 = property on="项目信息" class="Tbl (严格)"("Disabled"=w1782) -> ()  [unwired: 2 in, 2 out]
            n1290 = property on="产品编号" class="Str"("Disabled"=w1782) -> ()  [unwired: 2 in, 2 out]
            n1291 = Select(t=0, s=w1774, f=1) -> (s? t:f=w1773:i32)
            n1292 = property on="电池实际容量(A)" class="DigNum (严格)"("Disabled"=w1773) -> ()  [unwired: 2 in, 2 out]
            n1293 = property on="电池额定容量(A)" class="DigNum (严格)"("Disabled"=w1773) -> ()  [unwired: 2 in, 2 out]
            n1294 = property on="项目信息2" class="Clust (严格)"("DisabledEnum"=w1773) -> ()  [unwired: 2 in, 2 out]
            n1295 = global read "功能码全局.vi" "主板项目信息7"() -> (w1780:bool[])
            n1296 = Index Array(array=w1780, index #1=3 ("索引"), index #2=6 ("索引")) -> (element #1=w1778:bool, element #2=w1777:bool)
            n1297 = Not(x=w1784) -> (.not. x?=w1783:bool)
          }
          frame "配置文件版本" {
            w1797 = 2
            w1799 = FALSE
            n1298 = property on="使用者" class="DigNum (严格)"("Disabled"=w1797) -> ()  [unwired: 2 in, 2 out]
            n1299 = property on="SOH(%)" class="DigNum (严格)"("Disabled"=w1797) -> ()  [unwired: 2 in, 2 out]
            n1300 = property on="SOC(%)" class="DigNum (严格)"("Disabled"=w1797) -> ()  [unwired: 2 in, 2 out]
            n1301 = property on="电池实际容量(A)" class="DigNum (严格)"("Disabled"=w1797) -> ()  [unwired: 2 in, 2 out]
            n1302 = property on="从板个数" class="DigNum (严格)"("NumText.BGColor"=u32 13816530) -> ()  [unwired: 2 in, 2 out]
            n1303 = property on="电池额定容量(A)" class="DigNum (严格)"("Disabled"=w1797) -> ()  [unwired: 2 in, 2 out]
            n1304 = property on="系统时钟" class="Str"("Disabled"=w1797) -> ()  [unwired: 2 in, 2 out]
            n1305 = property on="车架(牌)号" class="Str"("Disabled"=w1797) -> ()  [unwired: 2 in, 2 out]
            n1306 = property on="项目信息" class="Tbl (严格)"("Disabled"=w1797) -> ()  [unwired: 2 in, 2 out]
            n1307 = property on="产品编号" class="Str"("Disabled"=w1797) -> ()  [unwired: 2 in, 2 out]
            n1308 = Select(t=0, s=w1788, f=1) -> (s? t:f=w1787:i32)
            n1309 = property on="项目信息2" class="Clust (严格)"("DisabledEnum"=w1787) -> ()  [unwired: 2 in, 2 out]
            n1310 = property on="配置文件版本" class="Str"("Disabled"=w1787) -> ()  [unwired: 2 in, 2 out]
            n1311 = global read "功能码全局.vi" "主板项目信息5"() -> (w1795:bool[])
            n1312 = global read "功能码全局.vi" "主板项目信息6"() -> (w1794:bool[])
            n1313 = Index Array(array=w1795, index=6 ("索引")) -> (element=w1792:bool)
            n1314 = Index Array(array=w1794, index=7 ("索引")) -> (element=w1791:bool)
            n1315 = Not(x=w1799) -> (.not. x?=w1798:bool)
          }
          frame "参数修改记录" {
            w1812 = 2
            w1814 = FALSE
            n1316 = property on="SOH(%)" class="DigNum (严格)"("Disabled"=w1812) -> ()  [unwired: 2 in, 2 out]
            n1317 = property on="SOC(%)" class="DigNum (严格)"("Disabled"=w1812) -> ()  [unwired: 2 in, 2 out]
            n1318 = property on="电池实际容量(A)" class="DigNum (严格)"("Disabled"=w1812) -> ()  [unwired: 2 in, 2 out]
            n1319 = property on="电池额定容量(A)" class="DigNum (严格)"("Disabled"=w1812) -> ()  [unwired: 2 in, 2 out]
            n1320 = property on="从板个数" class="DigNum (严格)"("NumText.BGColor"=u32 13816530) -> ()  [unwired: 2 in, 2 out]
            n1321 = property on="系统时钟" class="Str"("Disabled"=w1812) -> ()  [unwired: 2 in, 2 out]
            n1322 = property on="车架(牌)号" class="Str"("Disabled"=w1812) -> ()  [unwired: 2 in, 2 out]
            n1323 = property on="配置文件版本" class="Str"("Disabled"=w1812) -> ()  [unwired: 2 in, 2 out]
            n1324 = property on="项目信息" class="Tbl (严格)"("Disabled"=w1812) -> ()  [unwired: 2 in, 2 out]
            n1325 = property on="产品编号" class="Str"("Disabled"=w1812) -> ()  [unwired: 2 in, 2 out]
            n1326 = Select(t=0, s=w1803, f=1) -> (s? t:f=w1802:i32)
            n1327 = property on="使用者" class="DigNum (严格)"("Disabled"=w1802) -> ()  [unwired: 2 in, 2 out]
            n1328 = property on="项目信息2" class="Clust (严格)"("DisabledEnum"=w1802) -> ()  [unwired: 2 in, 2 out]
            n1329 = global read "功能码全局.vi" "主板项目信息7"() -> (w1809:bool[])
            n1330 = global read "功能码全局.vi" "主板项目信息5"() -> (w1810:bool[])
            n1331 = Index Array(array=w1809, index=0 ("索引")) -> (element=w1807:bool)
            n1332 = Index Array(array=w1810, index=7 ("索引")) -> (element=w1806:bool)
            n1333 = Not(x=w1814) -> (.not. x?=w1813:bool)
          }
          frame "车牌号" {
            w1827 = 2
            w1829 = FALSE
            n1334 = property on="SOH(%)" class="DigNum (严格)"("Disabled"=w1827) -> ()  [unwired: 2 in, 2 out]
            n1335 = property on="使用者" class="DigNum (严格)"("Disabled"=w1827) -> ()  [unwired: 2 in, 2 out]
            n1336 = property on="SOC(%)" class="DigNum (严格)"("Disabled"=w1827) -> ()  [unwired: 2 in, 2 out]
            n1337 = property on="电池实际容量(A)" class="DigNum (严格)"("Disabled"=w1827) -> ()  [unwired: 2 in, 2 out]
            n1338 = property on="电池额定容量(A)" class="DigNum (严格)"("Disabled"=w1827) -> ()  [unwired: 2 in, 2 out]
            n1339 = property on="从板个数" class="DigNum (严格)"("NumText.BGColor"=u32 13816530) -> ()  [unwired: 2 in, 2 out]
            n1340 = property on="系统时钟" class="Str"("Disabled"=w1827) -> ()  [unwired: 2 in, 2 out]
            n1341 = property on="配置文件版本" class="Str"("Disabled"=w1827) -> ()  [unwired: 2 in, 2 out]
            n1342 = property on="项目信息" class="Tbl (严格)"("Disabled"=w1827) -> ()  [unwired: 2 in, 2 out]
            n1343 = property on="产品编号" class="Str"("Disabled"=w1827) -> ()  [unwired: 2 in, 2 out]
            n1344 = Select(t=0, s=w1818, f=1) -> (s? t:f=w1817:i32)
            n1345 = property on="车架(牌)号" class="Str"("Disabled"=w1817) -> ()  [unwired: 2 in, 2 out]
            n1346 = property on="项目信息2" class="Clust (严格)"("DisabledEnum"=w1817) -> ()  [unwired: 2 in, 2 out]
            n1347 = global read "功能码全局.vi" "主板项目信息7"() -> (w1824:bool[])
            n1348 = global read "功能码全局.vi" "主板项目信息6"() -> (w1825:bool[])
            n1349 = Index Array(array=w1824, index=1 ("索引")) -> (element=w1822:bool)
            n1350 = Index Array(array=w1825, index=0 ("索引")) -> (element=w1821:bool)
            n1351 = Not(x=w1829) -> (.not. x?=w1828:bool)
          }
          frame "SOH" {
            w1841 = 2
            w1843 = FALSE
            n1352 = property on="使用者" class="DigNum (严格)"("Disabled"=w1841) -> ()  [unwired: 2 in, 2 out]
            n1353 = property on="SOC(%)" class="DigNum (严格)"("Disabled"=w1841) -> ()  [unwired: 2 in, 2 out]
            n1354 = property on="电池实际容量(A)" class="DigNum (严格)"("Disabled"=w1841) -> ()  [unwired: 2 in, 2 out]
            n1355 = property on="电池额定容量(A)" class="DigNum (严格)"("Disabled"=w1841) -> ()  [unwired: 2 in, 2 out]
            n1356 = property on="从板个数" class="DigNum (严格)"("NumText.BGColor"=u32 13816530) -> ()  [unwired: 2 in, 2 out]
            n1357 = property on="系统时钟" class="Str"("Disabled"=w1841) -> ()  [unwired: 2 in, 2 out]
